vi "Write Alarm Clocks.vi"() -> ()   [LabVIEW 2020]
uses:
  <vilib>/Utility/sysdir.llb/System Directory Type.ctl
  <vilib>/Utility/file.llb/Write Delimited Spreadsheet (string).vi
panel:
  out "Table Control":string[][](table)=[["# of Clocks", "Day", "Alarm time"], ["1", "5.05.2020", "07:30:00"], ["2", "5.05.2020", "08:00:00"], ["3", "5.05.2020", "08:30:00"], ["4", "5.05.2020", "09:00:00"], ["5", "5.05.2020", "09:30:00"], ["6", "5.05.2020", "10:00:00"], ["7", "5.05.2020", "10:30:00"], ["8", "5.05.2020", "11:00:00"], ["9", "5.05.2020", "11:30:00"], ["10", "5.05.2020", "12:00:00"], ["11", "5.05.2020", "12:30:00"], ["12", "5.05.2020", "13:00:00"], ["13", "5.05.2020", "13:30:00"], ["14", "5.05.2020", "14:00:00"], ["15", "5.05.2020", "14:30:00"], ["16", "5.05.2020", "15:00:00"], ["17", "5.05.2020", "15:30:00"], ["18", "5.05.2020", "16:00:00"], ["19", "5.05.2020", "16:30:00"], ["20", "5.05.2020", "17:00:00"]]
  in  "Interval (mins)":dbl=30.0
  in  "Time Stamp":timestamp=timestamp(3692318400 s since 1904-01-01) format="%<%X\n%x>T"
  in  "Number of Alarm Clocks":i32=20
  # "Please set the time that you want the clocks to start from(time stamp), interval between clock times and quantity of clocks."
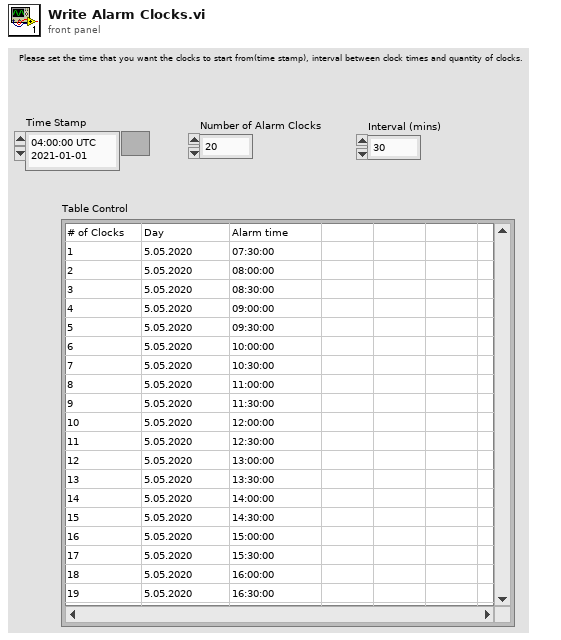
[diagram p1: front panel]
types:
  T1 = typedef "System Directory Type.ctl" = i32
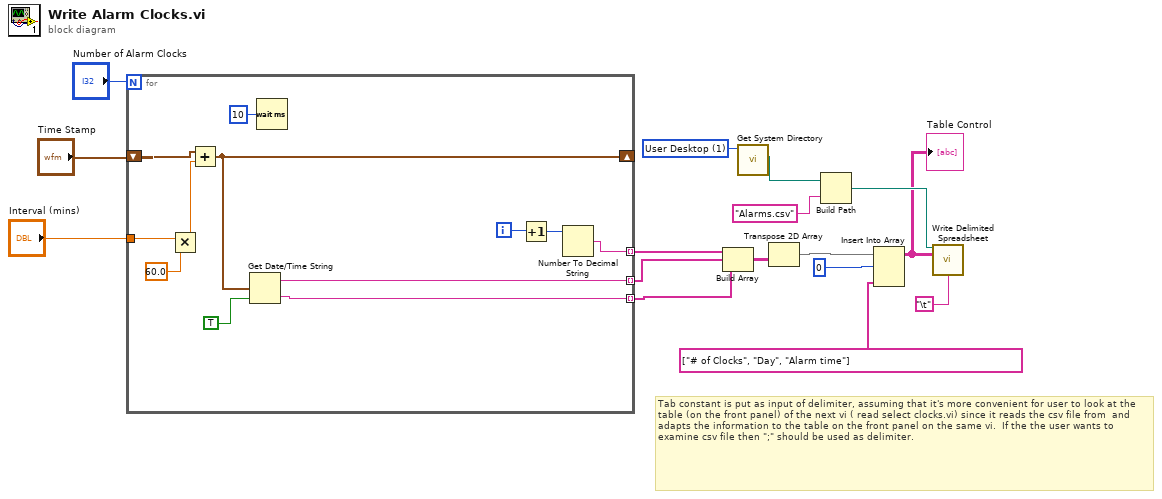
[diagram p0: block diagram]
diagram:
  w11 = T1 1 items=["User Home"=0, "User Desktop"=1, "User Documents"=2, "User Application Data"=3, "User Preferences"=4, "User Temporary"=5, "Public Documents"=6, "Public Application Data"=7, "Public Preferences"=8, "Public Cache"=13, "System Core Libraries"=9, "System Installed Libraries"=10, "Application Files"=11, "Boot Volume Root"=12] ("system directory type")
  # "Tab constant is put as input of delimiter, assuming that it's more convenient for user to look at the table (on the front panel) of the next vi ( read select clocks.vi) since it reads the csv file from  and adapts the information to the table on the front panel on the same vi.  If the the user wants to examine csv file then \";\" should be used as delimiter."
  n1 = for {
    N: "Number of Alarm Clocks" -> [_]
    shift-right: [w25] -> _
    shift-left: "Time Stamp" -> [w26]
    tunnel: [w24] -> w9 mode=indexing
    tunnel: "Interval (mins)" -> [w20]
    tunnel: [w18] -> w3 mode=indexing
    tunnel: [w17] -> w2 mode=indexing
    i -> [w22]
    n2 = Multiply(x=w20, y=60.0) -> (x*y=w19:dbl)
    n3 = Add(x=w26, y=w19) -> (x+y=w25:timestamp)
    n4 = Get Date/Time String(seconds (now)=w25, want seconds? (F)=TRUE) -> (date string=w17:string, time string=w18:string)  [unwired: 1 in]
    n5 = Wait (ms)(milliseconds to wait=u32 10) -> ()  [unwired: 1 out]
    n6 = Increment(x=w22) -> (x+1=w23:i32)
    n7 = Number To Decimal String(number=w23) -> (decimal integer string=w24:string)  [unwired: 1 in]
  }
  n8 = Build Array(w9, w2, w3) -> (w8:string[][])
  n9 = call <vilib>:"Get System Directory.vi"("system directory type"=w11) -> ("system directory"=w12:path)  [unwired: 10 in]
  n10 = Transpose 2D Array(2D array=w8) -> (transposed array=w7:string[][])
  n11 = Build Path(base path=w12, name or relative path="Alarms.csv") -> (appended path=w10:path)
  n12 = Insert Into Array(array=w7, index (row)=0, new element=string[] ["# of Clocks", "Day", "Alarm time"] ("new element/subarray")) -> (w4:string[][])  [unwired: 1 in]
  "Table Control" <- w4
  n13 = call-poly <vilib>:"Write Delimited Spreadsheet.vi"("file path (dialog if empty)"=w10, "2D data"=w4, "delimiter (\\t)"="\t") -> ()  [unwired: 11 in, 2 out]
